vi "Weigh Analyze.vi"(11 "Weigh":string) -> (0 "Weigh":string, 2 "标志位":string, 3 "Weigh":dbl)   [LabVIEW 2015]
panel:
  out "数组":string[](array[string])
  # "ST,NT,-  0.058 kg"
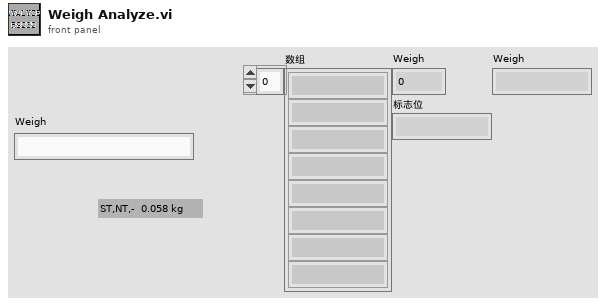
[diagram p1: front panel]
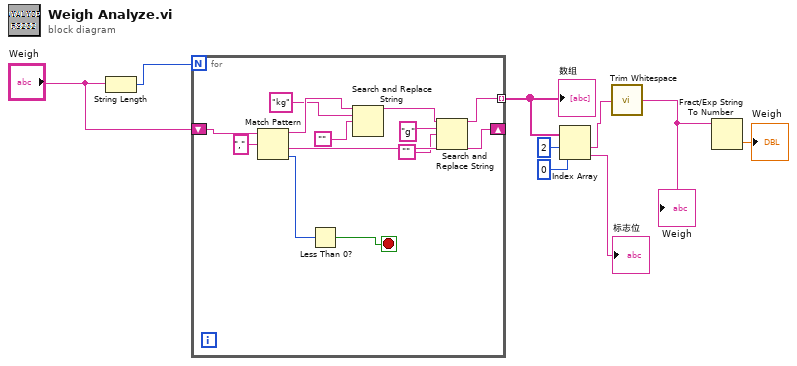
[diagram p0: block diagram]
diagram:
  n1 = String Length(string="Weigh") -> (length=w9:i32)
  n2 = for {
    N: w9 -> [_]
    shift-right: [w17] -> _
    shift-left: "Weigh" -> [w21]
    tunnel: [w12] -> w7 mode=indexing
    stop <- w18 stop-if-true
    n3 = Match Pattern(string=w21, regular expression="," ("正则表达式")) -> (before substring=w16:string, after substring=w17:string, offset past match=w19:i32)  [unwired: 1 in, 1 out]
    n4 = Less Than 0?(x=w19) -> (x < 0?=w18:bool)
    n5 = Search and Replace String(input string=w16, search string="kg" ("搜索字符串"), replace string="") -> (result string=w11:string)  [unwired: 5 in, 3 out]
    n6 = Search and Replace String(input string=w11, search string="g" ("搜索字符串"), replace string="") -> (result string=w12:string)  [unwired: 5 in, 3 out]
  }
  "数组" <- w7
  n7 = Index Array(array=w7, index #1=2 ("索引"), index #2=0 ("索引")) -> (element #1=w2:string, element #2=→"标志位":string)
  n8 = call <vilib>:"Trim Whitespace.vi"("string"=w2) -> ("trimmed string"=w1:string)  [unwired: 1 in]
  "Weigh" <- w1
  n9 = Fract/Exp String To Number(string=w1) -> (number=→"Weigh":dbl)  [unwired: 3 in, 1 out]
